vi "CalculateXYZ.vi"(3 "CMF":dbl[][](array[numeric]), 4 "Reflectance":dbl[](array[numeric]), 5 "Illuminant":dbl[](array[numeric])) -> (0 "Z":dbl, 1 "Y":dbl, 2 "X":dbl)   [LabVIEW 2014]
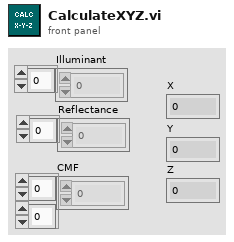
[diagram p1: front panel]
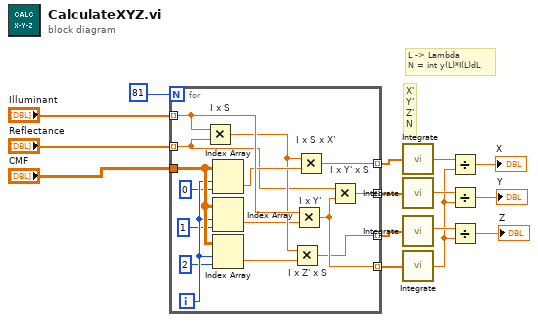
[diagram p0: block diagram]
diagram:
  # "X'\nY'\nZ'\nN"
  # "L -> Lambda\nN = int y(L)*I(L)dL"
  n1 = for {
    N: 81 -> [_]
    tunnel: "CMF" -> [w30]
    tunnel: "Illuminant" -> [w25] mode=indexing
    tunnel: "Reflectance" -> [w20] mode=indexing
    tunnel: [w19] -> w14 mode=indexing
    tunnel: [w18] -> w12 mode=indexing
    tunnel: [w17] -> w11 mode=indexing
    tunnel: [w16] -> w13 mode=indexing
    i -> [w29]
    n2 = Multiply "I x S"(x=w25, y=w20) -> (x*y=w22:dbl)
    n3 = Index Array(array=w30, index (row)=w29, index (col)=0 ("disabled index (col)")) -> (element=w24:dbl)
    n4 = Index Array(array=w30, index (row)=w29, index (col)=1 ("disabled index (col)")) -> (element=w21:dbl)
    n5 = Index Array(array=w30, index (row)=w29, index (col)=2 ("disabled index (col)")) -> (element=w23:dbl)
    n6 = Multiply "I x Z' x S"(x=w22, y=w23) -> (x*y=w16:dbl)
    n7 = Multiply "I x Y'"(x=w25, y=w21) -> (x*y=w19:dbl)
    n8 = Multiply "I x S x X'"(x=w22, y=w24) -> (x*y=w17:dbl)
    n9 = Multiply "I x Y' x S"(x=w20, y=w19) -> (x*y=w18:dbl)
  }
  n10 = call "Integrate.vi"("Array"=w11) -> ("Integral result"=w10:dbl)
  n11 = call "Integrate.vi"("Array"=w12) -> ("Integral result"=w9:dbl)
  n12 = call "Integrate.vi"("Array"=w13) -> ("Integral result"=w8:dbl)
  n13 = call "Integrate.vi"("Array"=w14) -> ("Integral result"=w7:dbl)
  n14 = Divide(x=w10, y=w7) -> (x/y=→"X":dbl)
  n15 = Divide(x=w9, y=w7) -> (x/y=→"Y":dbl)
  n16 = Divide(x=w8, y=w7) -> (x/y=→"Z":dbl)
